vi "Scale Module (Main) 1.vi"(10 "Config":variant, 11 "Main UI Message Queue":refnum<queue>) -> ()   [LabVIEW 2021]
doc: "This Continuous Measurement sample project is based on the Queued Message Handler template.\n\nThe Event Handling Loop generates messages based on user interface actions.\n\nThe Message Handling Loop processes messages generated by the Event Handling Loop, or by other messages. There are also Acquisition and Logging message handling loop subVIs, and a chart updating loop."
uses:
  support/Support Library.lvlib
  support/Message Queue/Enqueue Message (Single).vi
  <vilib>/ErrorRing/Error Ring.xnode
  controls/UI State.ctl
  <vilib>/Utility/error.llb/Error Cluster From Error Code.vi
  Measure Instrument/Scale Module Engine.lvlib
  Scale Module.lvlib
  <vilib>/Utility/miscctls.llb/LVPoint32TypeDef.ctl
  Scale Module Config Cluster.ctl
  Scale Module Settings Cluster.ctl
  Mettler Toledo/Controls/Settings Cluster.ctl
  Mettler Toledo/Mettler Toledo.lvlib
  Scale Module State Cluster.ctl
  Scale Module Display.ctl
  support/Message Queue/Message Cluster.ctl
panel:
  out "ScanCode":i16
  out "g":dbl
  in  "Settings Button":bool
  out "Log File path":path
  out "Status":string
  in  "Exit":bool
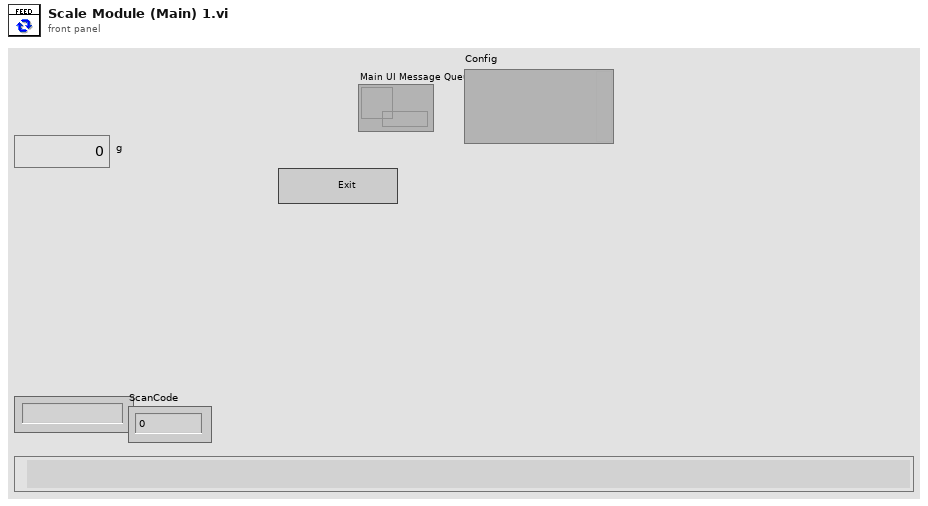
[diagram p1: front panel]
types:
  T1 = typedef "Scale Module.lvlib/Scale Module State Cluster.ctl" = cluster{"Scale Module Config":T2}
  T2 = typedef "Scale Module.lvlib/Scale Module Config Cluster.ctl" = cluster{"GUID":string, "Drop Coords":T3, "Process Name":string, "User name":string, "Queue Name":string, "Settings":T4, "Load Count":i32}
  T3 = typedef "LVPoint32TypeDef.ctl" = cluster{"Horizontal":i32, "Vertical":i32}
  T4 = typedef "Scale Module.lvlib/Scale Module Settings Cluster.ctl" = cluster{"Cycle Period":dbl, "Mettler":T5, "Scale Type":string}
  T5 = typedef "Mettler Toledo.lvlib/Settings Cluster.ctl" = cluster{"VISA resource name":refnum<visa-resource-name>, "Simulated?":bool}
  T6 = typedef "UI State.ctl" = enum16{"Idle", "Acquiring and Logging", "Waiting for Exit", "Waiting for Exit (Acq Stopped)", "Waiting for Exit (Log Stopped)", "Waiting for Stop", "Waiting for Stop (Acq Stopped)", "Waiting for Stop (Log Stopped)"}
  T7 = typedef "Message Queue.lvlib/All Message Queues.ctl" = cluster{"UI":refnum<queue>, "Engine":refnum<queue>, "Tempurature":refnum<queue>, "Temp Engine":refnum<queue>, "Pressure":refnum<queue>, "Pressure Engine":refnum<queue>, "FM Display":refnum<queue>, "OP Display":refnum<queue>, "Scale UI":refnum<queue>, "Scale Engine":refnum<queue>, "Scale Display":refnum<queue>}
  T8 = typedef "Scale Module.lvlib/Scale Module Display.ctl" = cluster{"Scale Value":dbl, "Cycle Period":dbl}
  T9 = cluster{"Shift":bool, "Ctrl":bool, "Alt":bool, "Cmd":bool, "Opt":bool}
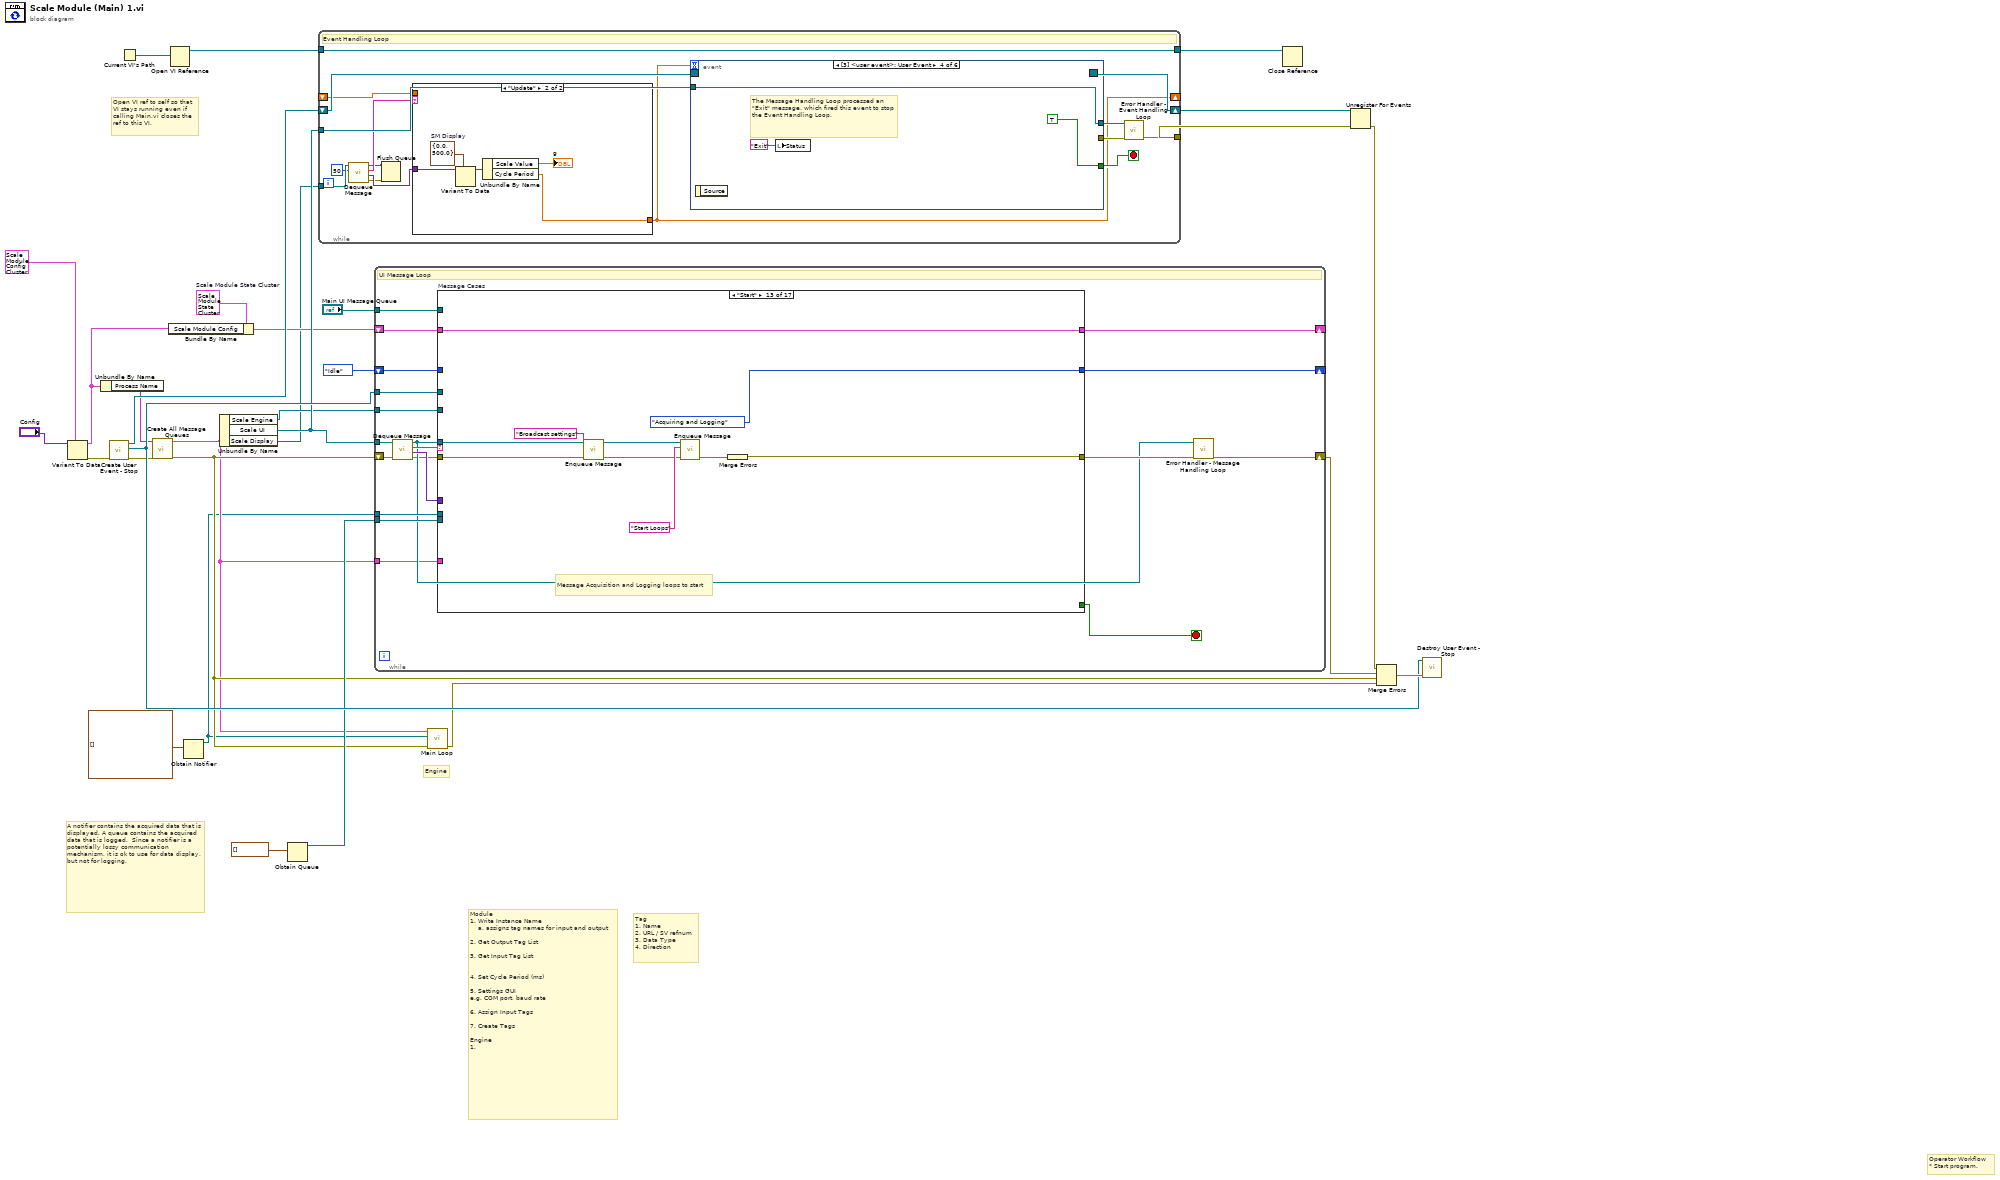
[diagram p0: block diagram]
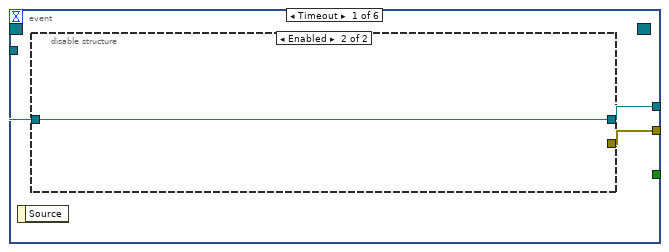
[diagram p3: hidden frame]
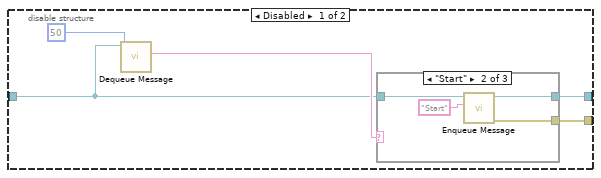
[diagram p4: hidden frame]
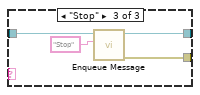
[diagram p6: hidden frame]
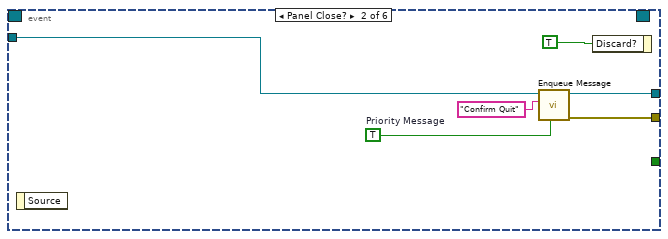
[diagram p7: hidden frame]
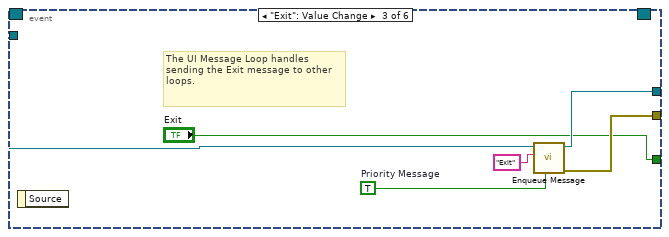
[diagram p8: hidden frame]
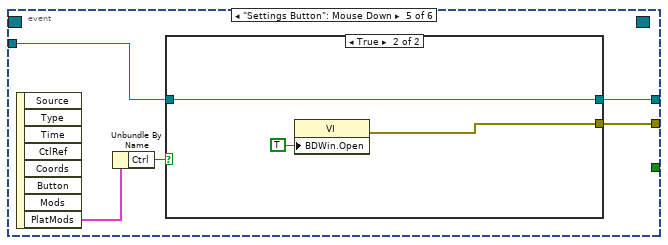
[diagram p9: hidden frame]
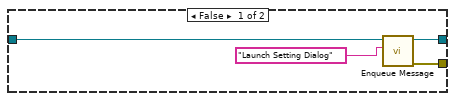
[diagram p10: hidden frame]
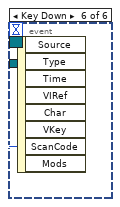
[diagram p11: hidden frame]
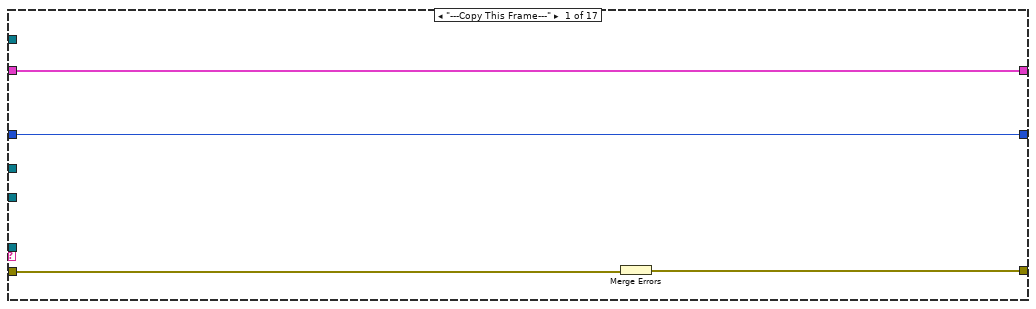
[diagram p12: hidden frame]
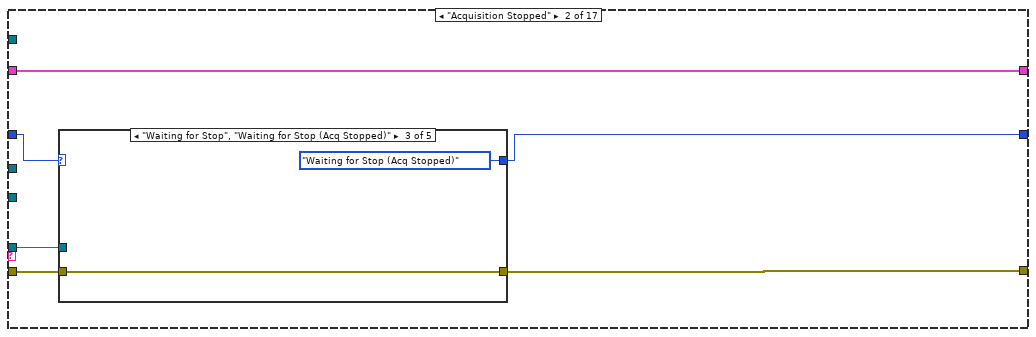
[diagram p13: hidden frame]
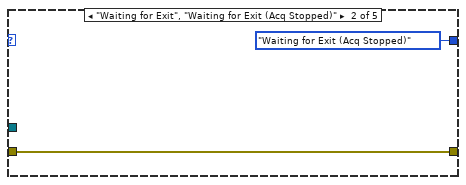
[diagram p15: hidden frame]
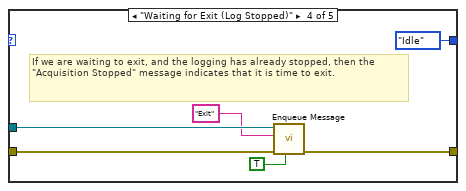
[diagram p16: hidden frame]
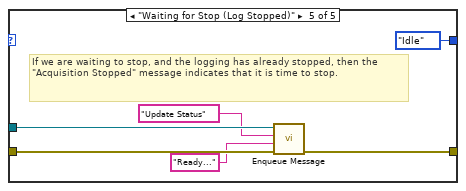
[diagram p17: hidden frame]
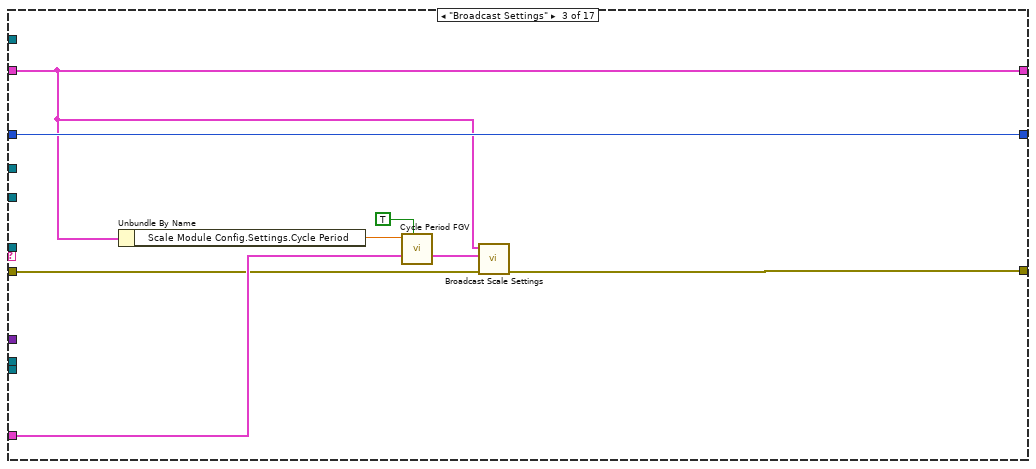
[diagram p18: hidden frame]
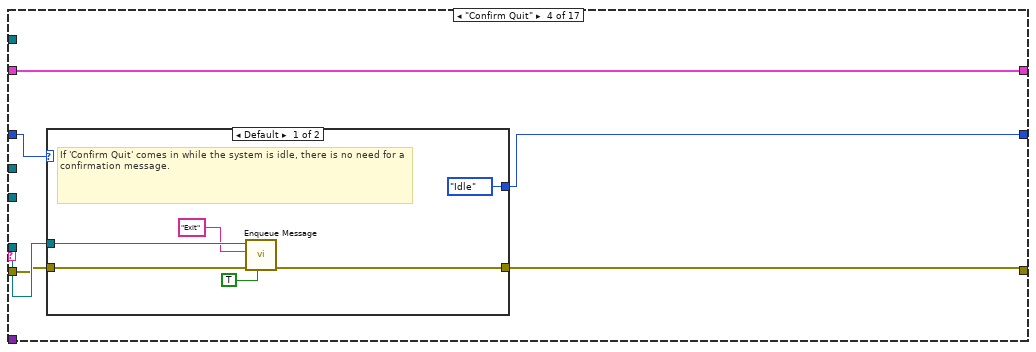
[diagram p19: hidden frame]
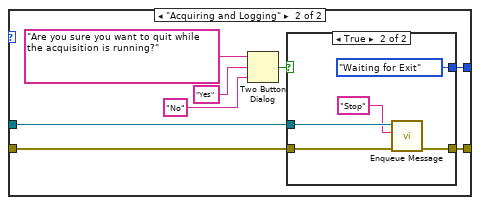
[diagram p20: hidden frame]
diagram:
  w3 = T1 {"Scale Module Config"={"GUID"="PID1-Mettler Toledo Scale 1", "Drop Coords"={"Horizontal"=0, "Vertical"=0}, "Process Name"="PID1-Setpoint", "User name"="", "Queue Name"="", "Settings"={"Cycle Period"=500.0, "Mettler"={"VISA resource name"="", "Simulated?"=FALSE}, "Scale Type"=""}, "Load Count"=0}}  # Scale Module State Cluster
  # "Open VI ref to self so that\nVI stays running even if\ncalling Main.vi closes the\nref to this VI."
  # "Engine"
  # "Operator Workflow\n* Start program."
  # "Module \n1. Write Instance Name\n    a. assigns tag names for input and output\n\n2. Get Output Tag List\n\n3. Get Input Tag List\n\n\n4. Set Cycle Period (ms)\n\n5. Settings GUI\ne.g. COM port, baud rate\n\n6. Assign Input Tags\n\n7. Create Tags\n\nEngine\n1."
  # "Tag\n1. Name\n2. URL / SV refnum\n3. Data Type\n4. Direction"
  # "A notifier contains the acquired data that is displayed. A queue contains the acquired data that is logged.  Since a notifier is a potentially lossy communication mechanism, it is ok to use for data display, but not for logging."
  n1 = Variant To Data(type=T2 {"GUID"="", "Drop Coords"={"Horizontal"=0, "Vertical"=0}, "Process Name"="", "User name"="", "Queue Name"="", "Settings"={"Cycle Period"=500.0, "Mettler"={"VISA resource name"="", "Simulated?"=FALSE}, "Scale Type"=""}, "Load Count"=0} ("Feed Module Config"), Variant="Config") -> (data=w1:T2, error out=w7:errorcluster)  [unwired: 1 in]
  n2 = Unbundle By Name(w1) -> ("Process Name"=w6:string)
  n3 = call "Create User Event - Stop.vi"("error in (no error)"=w7) -> ("error out"=w25:errorcluster, "User Event - Stop"=w26:refnum<user-event>, "Stop Event Registration Refnum"=w27:refnum<event-registration>)  [unwired: 8 in]
  n4 = Current VI's Path() -> (path=w10:path)
  n5 = call "Create All Message Queues.vi"("error in (no error)"=w25, "Process Name"=w6) -> ("error out"=w15:errorcluster, "Message Queues out"=w14:T7)  [unwired: 8 in]
  n6 = Bundle By Name(cluster=w3, "Scale Module Config"=w1) -> (w8:T1)
  n7 = Open VI Reference(vi path=w10) -> (vi reference=w11:refnum<vi>)  [unwired: 5 in, 1 out]
  n8 = Obtain Notifier(notification data type=waveform(dbl)[] []) -> (notifier out=w13:refnum<notifier>)  [unwired: 3 in, 2 out]
  n9 = Unbundle By Name(w14) -> ("Scale Engine"=w18:refnum<queue>, "Scale UI"=w22:refnum<queue>, "Scale Display"=w2:refnum<queue>)
  n10 = Obtain Queue(element data type=waveform(dbl)[] []) -> (queue out=w17:refnum<queue>)  [unwired: 4 in, 2 out]
  n11 = while {
    tunnel: w22 -> [w40]
    tunnel: [w42] -> w29
    shift-right: [w41] -> w23
    shift-left: w27 -> [w46]
    tunnel: [w39] -> w12
    tunnel: w11 -> [w39]
    tunnel: w2 -> [w38]
    shift-right: [w35] -> _
    shift-left: _ -> [w34]
    stop <- w45 stop-if-true
    # "Event Handling Loop"
    n12 = call "Dequeue Message.vi"("timeout in ms (-1)"=50, "Message Queue"=w38) -> ("error out"=w31:errorcluster, "Message Data"=w36:variant, "Message"=w37:string, "dup Message Queue"=w32:refnum<queue>)  [unwired: 6 in]
    n13 = Flush Queue(queue=w32, error in (no error)=w31) -> ()  [unwired: 3 out]
    n14 = case shown="\"Update\"" w37 {
      tunnel: w36 -> [_ w52]
      tunnel: [w47 w49] -> w35
      tunnel: w34 -> [w47 _]
      frame "False", Default {
      }
      frame "Update" {
        w48 = T8 {"Scale Value"=0.0, "Cycle Period"=500.0}  # SM Display
        n15 = Variant To Data(type=w48, Variant=w52) -> (data=w51:T8)  [unwired: 1 in, 1 out]
        n16 = Unbundle By Name(w51) -> ("Scale Value"=→"g":dbl, "Cycle Period"=w49:dbl)
      }
    }
    n17 = event shown="[3] <user event>: User Event" {
      selector: w46 -> [_ _ _ _ _ _]
      dyn-events: [_ _ _ _ _ _] -> w41
      timeout: w35 -> [_ _ _ _ _ _]
      tunnel: [_ _ "Exit" TRUE ("Discard?") _ _] -> w45
      tunnel: w40 -> [w55 w72 w78 w82 w87 _]
      tunnel: [w53 w70 w81 _ w89 _] -> w43
      tunnel: [w54 w71 w77 w82 w88 _] -> w44
      event Timeout {
        n18 = event-data() -> ()  [unwired: 1 in, 1 out]
        n19 = disable-structure shown="Enabled" {
          disable-tunnel: w55 -> [w58 w69]
          disable-tunnel: [w57 w69] -> w54
          disable-tunnel: [w56 _] -> w53
          frame Disabled {
            n20 = call "Dequeue Message.vi"("timeout in ms (-1)"=50, "Message Queue"=w58) -> ("Message"=w59:string)  [unwired: 6 in, 3 out]
            n21 = case shown="\"Start\"" w59 {
              tunnel: w58 -> [_ w63 w67]
              tunnel: [_ w62 w66] -> w57
              tunnel: [_ w61 w65] -> w56
              frame "None", Default {
              }
              frame "Start" {
                n22 = call-poly "Enqueue Message.vi"("Message"="Start", "Message Queue"=w63) -> ("error out"=w61:errorcluster, "dup Message Queue"=w62:refnum<queue>)  [unwired: 8 in]
              }
              frame "Stop" {
                n23 = call-poly "Enqueue Message.vi"("Message"="Stop", "Message Queue"=w67) -> ("error out"=w65:errorcluster, "dup Message Queue"=w66:refnum<queue>)  [unwired: 8 in]
              }
            }
          }
          frame Enabled {
          }
        }
      }
      event Panel Close? {
        w73 = TRUE  # Priority Message
        n24 = event-data() -> ()  [unwired: 1 in, 1 out]
        n25 = call-poly "Enqueue Message.vi"("Priority Message? (F)"=w73, "Message"="Confirm Quit", "Message Queue"=w72) -> ("error out"=w70:errorcluster, "dup Message Queue"=w71:refnum<queue>)  [unwired: 7 in]
        n26 = event-data("Discard?"=TRUE) -> ()  [unwired: 1 in, 1 out]
      }
      event "Exit": Value Change {
        w79 = TRUE  # Priority Message
        # "The UI Message Loop handles sending the Exit message to other loops."
        n27 = event-data() -> ()  [unwired: 1 in, 1 out]
        n28 = call-poly "Enqueue Message.vi"("Priority Message? (F)"=w79, "Message"="Exit", "Message Queue"=w78) -> ("error out"=w81:errorcluster, "dup Message Queue"=w77:refnum<queue>)  [unwired: 7 in]
      }
      event User Event {
        # "The Message Handling Loop processed an \"Exit\" message, which fired this event to stop the Event Handling Loop."
        n29 = event-data() -> ()  [unwired: 1 in, 1 out]
        n30 = local write "Status"("Exit" ("Exit String")) -> ()
      }
      event "Settings Button": Mouse Down {
        n31 = event-data() -> ("PlatMods"=w86:T9)  [unwired: 1 in, 7 out]
        n32 = Unbundle By Name(w86) -> ("Ctrl"=w85:bool)
        n33 = case shown="True" w85 {
          tunnel: [w93 w94] -> w89
          tunnel: [w92 w95] -> w88
          tunnel: w87 -> [w91 w95]
          frame False {
            n34 = call-poly "Enqueue Message.vi"("Message"="Launch Setting Dialog", "Message Queue"=w91) -> ("error out"=w93:errorcluster, "dup Message Queue"=w92:refnum<queue>)  [unwired: 8 in]
          }
          frame True {
            n35 = property class="VI"("BDWin.Open"=TRUE ("Block Diagram Window:Open")) -> (error out=w94:errorcluster)  [unwired: 2 in, 1 out]
          }
        }
      }
      event Key Down {
        n36 = event-data() -> ("ScanCode"=→"ScanCode":i16)  [unwired: 1 in, 7 out]
      }
    }
    n37 = call "Error Handler - Event Handling Loop.vi"("error in (no error)"=w43, "Message Queue"=w44) -> ("dup error in"=w42:errorcluster)  [unwired: 8 in, 1 out]
  }
  n38 = while {
    tunnel: w22 -> [w111]
    tunnel: w26 -> [w115]
    shift-right: [w107] -> w30
    shift-left: w15 -> [w114]
    shift-right: [w98] -> _
    shift-left: w8 -> [w100]
    tunnel: w13 -> [w110]
    tunnel: w17 -> [w109]
    shift-right: [w104] -> _
    shift-left: UI_State."Idle" ("UI State") -> [w105]
    tunnel: w18 -> [w103]
    tunnel: w14 -> [w102]
    tunnel: "Main UI Message Queue" -> [w99]
    stop <- w116 stop-if-true
    # "UI Message Loop"
    n39 = call "Dequeue Message.vi"("error in (no error)"=w114, "Message Queue"=w111) -> ("error out"=w101:errorcluster, "Message Data"=w112:variant, "Message"=w113:string, "dup Message Queue"=w106:refnum<queue>)  [unwired: 6 in]
    n40 = case "Message Cases" shown="\"Start\"" w113 {
      selector: w113 -> [_ _ _ _ _ _ _ _ _ _ _ _ _ _ _ _ w345]
      tunnel: w106 -> [_ w122 _ w156 _ w196 w207 w221 _ w240 w254 w275 w301 _ w331 _ _]
      tunnel: w101 -> [w120 w124 w146 w155 w181 w187 w211 w224 w234 w236 w250 w277 w299 w310 w326 w341 _]
      tunnel: [w119 w123 w151 w154 w182 w197 w202 w225 w234 w245 w261 w276 w307 w315 w332 w342 w346] -> w108
      tunnel: [_ _ _ _ _ _ _ TRUE _ _ _ _ _ _ _ _ _] -> w116
      tunnel: w112 -> [_ _ _ _ w184 _ w210 _ _ _ _ _ _ _ _ w340 _]
      tunnel: w115 -> [_ _ _ _ _ _ _ w223 _ _ _ _ _ _ _ _ _]
      tunnel: w100 -> [w117 w121 w145 w152 w179 w186 w200 w212 w231 w235 w256 w274 w298 w308 w321 w335 w343]
      tunnel: w110 -> [_ _ _ _ _ _ _ w220 _ _ _ _ _ _ _ _ _]
      tunnel: w109 -> [_ _ _ _ _ _ _ w216 _ _ _ _ _ _ _ _ _]
      tunnel: w105 -> [w118 w126 w150 w157 w180 w192 w201 _ _ _ w260 w279 _ _ w327 w336 w344]
      tunnel: [w118 w125 w150 w153 w180 w193 w201 UI_State."Idle" ("UI State") UI_State."Idle" ("UI State") UI_State."Idle" ("UI State") w260 w278 UI_State."Acquiring and Logging" ("UI State") UI_State."Acquiring and Logging" ("UI State") w328 w336 w344] -> w104
      tunnel: w103 -> [_ _ _ _ _ w191 _ w214 _ _ _ _ _ w313 w325 _ _]
      tunnel: w102 -> [_ _ w149 _ _ _ _ _ _ _ _ _ _ _ _ _ _]
      tunnel: w99 -> [_ _ _ _ _ _ _ _ _ _ w257 _ _ _ _ _ _]
      tunnel: [w117 w121 w145 w152 w179 w186 w200 w212 w231 w235 w248 w274 w298 w308 w321 w335 w343] -> w98
      frame "---Copy This Frame---" {
        # "Duplicate this frame when creating new messages.  Change this comment in the duplicated frame to describe this message."
        n41 = Merge Errors(w120) -> (w119:errorcluster)
      }
      frame "Acquisition Stopped" {
        # "Logic for determining what action to take when the acquisition has stopped."
        n42 = case shown="\"Waiting for Stop\", \"Waiting for Stop (Acq Stopped)\"" w126 {
          selector: w126 -> [w128 _ _ _ _]
          tunnel: [w128 UI_State."Waiting for Exit (Acq Stopped)" ("UI State") UI_State."Waiting for Stop (Acq Stopped)" ("UI State") UI_State."Idle" ("UI State") UI_State."Idle" ("UI State")] -> w125
          tunnel: w124 -> [w127 w129 w131 w137 w143]
          tunnel: [w127 w129 w131 w136 w142] -> w123
          tunnel: w122 -> [_ _ _ w135 w141]
          frame Default {
          }
          frame "Waiting for Exit", "Waiting for Exit (Acq Stopped)" {
          }
          frame "Waiting for Stop", "Waiting for Stop (Acq Stopped)" {
          }
          frame "Waiting for Exit (Log Stopped)" {
            # "If we are waiting to exit, and the logging has already stopped, then the \"Acquisition Stopped\" message indicates that it is time to exit."
            n43 = call-poly "Enqueue Message.vi"("Priority Message? (F)"=TRUE, "error in (no error)"=w137, "Message"="Exit", "Message Queue"=w135) -> ("error out"=w136:errorcluster)  [unwired: 6 in, 1 out]
          }
          frame "Waiting for Stop (Log Stopped)" {
            # "If we are waiting to stop, and the logging has already stopped, then the \"Acquisition Stopped\" message indicates that it is time to stop."
            n44 = call-poly "Enqueue Message.vi"("error in (no error)"=w143, "Message Data"="Ready..." ("Message"), "Message"="Update Status", "Message Queue"=w141) -> ("error out"=w142:errorcluster)  [unwired: 6 in, 1 out]
          }
        }
      }
      frame "Broadcast Settings" {
        # "Send the 'Update Settings' message to the Logging and Acquisition message loops."
        n45 = Unbundle By Name(w145) -> ("Scale Module Config.Settings.Cycle Period"=w147:dbl)
        n46 = call "Cycle Period FGV.vi"("Write"=TRUE, "Cycle Period In (ms)"=w147) -> ()  [unwired: 8 in, 2 out]
        n47 = call "Broadcast Scale Settings.vi"("error in (no error)"=w146, "Message Queues"=w149, "Scale Module Config"=w145) -> ("error out"=w151:errorcluster)  [unwired: 8 in]
      }
      frame "Confirm Quit" {
        # "Confirm Quit - Message that can confirm whether or not the user wants to exit the application."
        n48 = case shown="Default" w157 {
          tunnel: w156 -> [w162 w168]
          tunnel: w155 -> [w161 w166]
          tunnel: [w158 w165] -> w154
          tunnel: [UI_State."Idle" ("UI State") w164] -> w153
          frame Default {
            # "If 'Confirm Quit' comes in while the system is idle, there is no need for a confirmation message."
            n49 = call-poly "Enqueue Message.vi"("Priority Message? (F)"=TRUE, "error in (no error)"=w161, "Message"="Exit", "Message Queue"=w162) -> ("error out"=w158:errorcluster)  [unwired: 6 in, 1 out]
          }
          frame "Acquiring and Logging" {
            n50 = Two Button Dialog(message="Are you sure you want to quit while the acquisition is running?" ("Confirm Quit Message"), 1:"No" ("No"), 2:"Yes" ("Yes")) -> (T button?=w167:bool)
            n51 = case shown="True" w167 {
              tunnel: w168 -> [_ w178]
              tunnel: w166 -> [w172 w177]
              tunnel: [w172 w176] -> w165
              tunnel: [UI_State."Acquiring and Logging" ("UI State") UI_State."Waiting for Exit" ("UI State")] -> w164
              frame False {
                # "User did not want to quit."
              }
              frame True {
                n52 = call-poly "Enqueue Message.vi"("error in (no error)"=w177, "Message"="Stop", "Message Queue"=w178) -> ("error out"=w176:errorcluster)  [unwired: 7 in, 1 out]
              }
            }
          }
        }
      }
      frame "Display Log File Path" {
        n53 = Variant To Data(error in=w181, type=path "", Variant=w184) -> (data=→"Log File path":path, error out=w182:errorcluster)
      }
      frame "E-Stop" {
        # "Message Acquisition and Logging loops to stop"
        # "Stop the pumps."
        n54 = call-poly "Enqueue Message.vi"("error in (no error)"=w187, "Message Data"="Ready..." ("Ready..."), "Message"="Update Status", "Message Queue"=w196) -> ("error out"=w189:errorcluster)  [unwired: 6 in, 1 out]
        n55 = call-poly "Enqueue Message.vi"("error in (no error)"=w189, "Message"="Stop", "Message Queue"=w191) -> ("error out"=w188:errorcluster)  [unwired: 7 in, 1 out]
        n56 = case shown="\"Waiting for Exit\"" w192 {
          selector: w192 -> [_ w199]
          tunnel: [UI_State."Waiting for Stop" ("UI State") w199] -> w193
          frame Default {
          }
          frame "Waiting for Exit" {
          }
        }
        n57 = Merge Errors(w188) -> (w197:errorcluster)
      }
      frame "Error" {
        # "Error - Check the error message data and respond accordingly. This message is sent by the \"Error Handler\" VIs at the end of each loop in this application."
        n58 = Variant To Data(error in=w211, type=errorcluster {"status"=FALSE, "code"=0, "source"=""} ("error out"), Variant=w210) -> (data=w208:errorcluster, error out=w204:errorcluster)
        n59 = call <vilib>:"Simple Error Handler.vi"("error in (no error)"=w208) -> ()  [unwired: 4 in, 5 out]
        n60 = call-poly "Enqueue Message.vi"("Priority Message? (F)"=TRUE, "Message"="Exit", "Message Queue"=w207) -> ("error out"=w203:errorcluster)  [unwired: 7 in, 1 out]
        n61 = Merge Errors(w203, w204) -> (w202:errorcluster)
      }
      frame "Exit" {
        # "Don't check the error outs. The acquisition and logging queues may have already been released."
        # "Close references owned by the Main VI."
        # "Stop the VI"
        # "Exit - Fire the User Event to stop the Event Handling Loop.  Also send Exit messages to the Acquisition and Logging loops."
        n62 = Release Queue(queue=w221, error in (no error)=w224) -> (error out=w219:errorcluster)  [unwired: 1 in, 2 out]
        n63 = call "Fire User Event - Stop.vi"("User Event - Stop"=w223) -> ("error out"=w222:errorcluster)  [unwired: 10 in]
        n64 = Release Notifier(notifier=w220, error in (no error)=w219) -> (error out=w218:errorcluster)  [unwired: 1 in, 2 out]
        n65 = Build Array(w214) -> (w213:refnum<queue>[])
        n66 = Release Queue(queue=w216, error in (no error)=w218) -> (error out=w217:errorcluster)  [unwired: 1 in, 2 out]
        n67 = for {
          tunnel: w213 -> [w228] mode=indexing
          n68 = call-poly "Enqueue Message.vi"("Message"="Stop", "Message Queue"=w228) -> ("dup Message Queue"=w229:refnum<queue>)  [unwired: 8 in, 1 out]
          n69 = call-poly "Enqueue Message.vi"("Message"="Exit", "Message Queue"=w229) -> ()  [unwired: 8 in, 2 out]
        }
        n70 = Merge Errors(w222, w217) -> (w225:errorcluster)
      }
      frame "Init UI Refs" {
        # "Init UI Refs - Store control references for UI controls.  Also enable/disable controls appropriately."
        n71 = property class="VI"("Front Panel.Closeable"=TRUE ("Front Panel Window:Closeable")) -> ()  [unwired: 2 in, 2 out]
      }
      frame "Initialize" {
        # "Initialize - Get configuration settings, then message the UI to initialize, and broadcast the settings to the other message loops."
        n72 = call-poly "Enqueue Message.vi"("error in (no error)"=w236, "Message"="Init UI Refs", "Message Queue"=w240) -> ("error out"=w238:errorcluster, "dup Message Queue"=w239:refnum<queue>)  [unwired: 7 in]
        n73 = call-poly "Enqueue Message.vi"("error in (no error)"=w238, "Message"="Broadcast Settings", "Message Queue"=w239) -> ("error out"=w247:errorcluster, "dup Message Queue"=w246:refnum<queue>)  [unwired: 7 in]
        n74 = call-poly "Enqueue Message.vi"("error in (no error)"=w247, "Message Data"="Ready..." ("Ready..."), "Message"="Update Status", "Message Queue"=w246) -> ("error out"=w245:errorcluster)  [unwired: 6 in, 1 out]
      }
      frame "Launch Settings Dialog" {
        # "Launch the Settings Dialog when the user clicks the 'Settings' button."
        n75 = Unbundle By Name(w256) -> ("Scale Module Config"=w255:T2)
        n76 = Unbundle By Name(w255) -> ("Load Count"=w258:i32)
        n77 = Increment(x=w258) -> (x+1=w259:i32)
        n78 = Bundle By Name(cluster=w255, "Load Count"=w259) -> (w253:T2)
        n79 = call "Scale Settings Dialog.vi"("error in (no error)"=w250, "Scale Module Config In"=w253) -> ("error out"=w251:errorcluster, "UI Refresh Needed?"=w249:bool, "Scale Module Config Out"=w252:T2)  [unwired: 6 in, 1 out]
        n80 = case shown="False" w249 {
          tunnel: w251 -> [w272 w273]
          tunnel: [w269 w273] -> w261
          tunnel: w257 -> [w270 _]
          tunnel: w254 -> [w267 _]
          frame False {
            n81 = call-poly "Enqueue Message.vi"("error in (no error)"=w272, "Message"="Broadcast Settings", "Message Queue"=w267) -> ("error out"=w263:errorcluster, "dup Message Queue"=w264:refnum<queue>)  [unwired: 7 in]
            n82 = call-poly "Enqueue Message.vi"("error in (no error)"=w263, "Message"="Start", "Message Queue"=w264) -> ("error out"=w262:errorcluster)  [unwired: 7 in, 1 out]
            n83 = call-poly "Enqueue Message.vi"("error in (no error)"=w272, "Message"="Save Config (Scale Module)", "Message Queue"=w270) -> ("error out"=w268:errorcluster)  [unwired: 7 in, 1 out]
            n84 = Merge Errors(w268, w262) -> (w269:errorcluster)
          }
          frame True {
          }
        }
        n85 = Bundle By Name(cluster=w256, "Scale Module Config"=w252) -> (w248:T1)
      }
      frame "Logging Stopped" {
        # "Logic for determining what action to take when the logging has stopped."
        n86 = case shown="\"Waiting for Exit (Acq Stopped)\"" w279 {
          selector: w279 -> [w281 _ _ _ _]
          tunnel: [w281 UI_State."Waiting for Exit (Log Stopped)" ("UI State") UI_State."Waiting for Stop (Log Stopped)" ("UI State") UI_State."Idle" ("UI State") UI_State."Idle" ("UI State")] -> w278
          tunnel: w277 -> [w280 w282 w284 w290 w296]
          tunnel: [w280 w282 w284 w289 w295] -> w276
          tunnel: w275 -> [_ _ _ w288 w294]
          frame Default {
          }
          frame "Waiting for Exit", "Waiting for Exit (Log Stopped)" {
          }
          frame "Waiting for Stop", "Waiting for Stop (Log Stopped)" {
          }
          frame "Waiting for Exit (Acq Stopped)" {
            # "If we are waiting to exit, and the acquisition has already stopped, then the \"Logging Stopped\" message indicates that it is time to exit."
            n87 = call-poly "Enqueue Message.vi"("Priority Message? (F)"=TRUE, "error in (no error)"=w290, "Message"="Exit", "Message Queue"=w288) -> ("error out"=w289:errorcluster)  [unwired: 6 in, 1 out]
          }
          frame "Waiting for Stop (Acq Stopped)" {
            # "If we are waiting to stop, and the acquisition has already stopped, then the \"Logging Stopped\" message indicates that it is time to stop."
            n88 = call-poly "Enqueue Message.vi"("error in (no error)"=w296, "Message Data"="Ready..." ("Message"), "Message"="Update Status", "Message Queue"=w294) -> ("error out"=w295:errorcluster)  [unwired: 6 in, 1 out]
          }
        }
      }
      frame "Start" {
        # "Message Acquisition and Logging loops to start"
        # "Start - Enable/Disable buttons appropriately for an acquisition that has started, and update status display."
        n89 = call-poly "Enqueue Message.vi"("error in (no error)"=w299, "Message"="Broadcast settings", "Message Queue"=w301) -> ("error out"=w302:errorcluster, "dup Message Queue"=w300:refnum<queue>)  [unwired: 7 in]
        n90 = call-poly "Enqueue Message.vi"("error in (no error)"=w302, "Message"="Start Loops", "Message Queue"=w300) -> ("error out"=w303:errorcluster)  [unwired: 7 in, 1 out]
        n91 = Merge Errors(w303) -> (w307:errorcluster)
      }
      frame "Start Loops" {
        # "Message Acquisition and Logging loops to start"
        # "Start - Enable/Disable buttons appropriately for an acquisition that has started, and update status display."
        n92 = Unbundle By Name(w308) -> ("Scale Module Config.Process Name"=w309:string)
        n93 = Build Array(w313) -> (w311:refnum<queue>[])
        n94 = for {
          tunnel: w310 -> [w319]
          tunnel: [w318] -> w312 mode=indexing
          tunnel: w311 -> [w317] mode=indexing
          tunnel: w309 -> [w316]
          n95 = call-poly "Enqueue Message.vi"("error in (no error)"=w319, "Message Data"=w316, "Message"="Start", "Message Queue"=w317) -> ("error out"=w318:errorcluster)  [unwired: 6 in, 1 out]
        }
        n96 = property class="VI"("Front Panel.Title"=w309) -> ()  [unwired: 2 in, 2 out]
        n97 = Merge Errors(w312) -> (w315:errorcluster)
      }
      frame "Stop" {
        # "Stop - Enable/Disable buttons appropriately for an acquisition that has stopped, and update status display."
        n98 = call-poly "Enqueue Message.vi"("error in (no error)"=w326, "Message Data"="Ready..." ("Ready..."), "Message"="Update Status", "Message Queue"=w331) -> ("error out"=w324:errorcluster)  [unwired: 6 in, 1 out]
        n99 = call-poly "Enqueue Message.vi"("error in (no error)"=w324, "Message"="Stop", "Message Queue"=w325) -> ("error out"=w322:errorcluster)  [unwired: 7 in, 1 out]
        n100 = case shown="\"Waiting for Exit\"" w327 {
          selector: w327 -> [_ w334]
          tunnel: [UI_State."Waiting for Stop" ("UI State") w334] -> w328
          frame Default {
          }
          frame "Waiting for Exit" {
          }
        }
        n101 = Merge Errors(w322) -> (w332:errorcluster)
      }
      frame "Update Status" {
        # "Update Display - Convert the message data to a string to display in the Status indicator."
        n102 = Variant To Data(error in=w341, type="", Variant=w340) -> (data=→"Status":string, error out=w338:errorcluster)
        n103 = Merge Errors(w338) -> (w342:errorcluster)
      }
      frame Default {
        # "'Default' case only runs if there is a message that isn't defined in any of the other cases.  Output a programming error."
        n104 = xnode "Error Ring"("parameter 0"=w345) -> ("error out"=w346:errorcluster)
      }
    }
    n105 = call "Error Handler - Message Handling Loop.vi"("error in (no error)"=w108, "Message Queue"=w106) -> ("dup error in"=w107:errorcluster)  [unwired: 8 in, 1 out]
  }
  n106 = call "Main Loop.vi"("error in (no error)"=w15, "Chart Notifier"=w13, "Message Queues"=w14) -> ("error out"=w16:errorcluster)  [unwired: 8 in]
  n107 = Close Reference(reference=w12) -> ()  [unwired: 1 in, 1 out]
  n108 = Unregister For Events(event registration refnum=w23, error in=w29) -> (error out=w24:errorcluster)
  n109 = Merge Errors(w24, w30, w15, w16) -> (w28:errorcluster)
  n110 = call "Destroy User Event - Stop.vi"("error in (no error)"=w28, "User Event - Stop"=w26) -> ()  [unwired: 9 in, 1 out]
